vi "uw2up.vi"(2 "error in (no error)":errorcluster, 3 "uw":dbl) -> (0 "error out":errorcluster, 1 "up":dbl)   [LabVIEW 2021]
panel:
  out "a":dbl=0.0696
  out "b":dbl=-64.3266
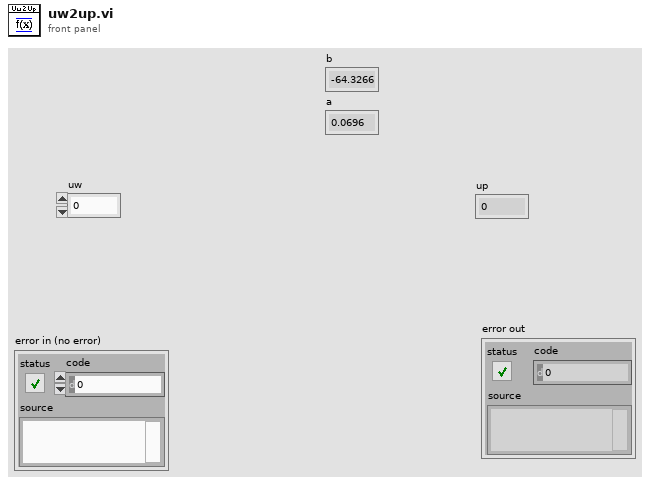
[diagram p1: front panel]
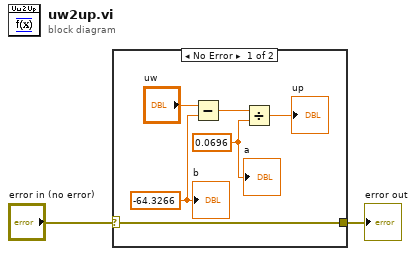
[diagram p0: block diagram]
diagram:
  n1 = case shown="No Error" "error in (no error)" {
    selector: "error in (no error)" -> [w8 w9]
    tunnel: [w8 w9] -> w1
    frame No Error {
      w4 = 0.0696 ("y")
      w6 = -64.3266 ("y")
      n2 = Subtract(x="uw", y=w6) -> (x-y=w5:dbl)
      n3 = Divide(x=w5, y=w4) -> (x/y=→"up":dbl)
      "b" <- w6
      "a" <- w4
    }
    frame Error {
    }
  }
  "error out" <- w1
